vi "Get variant data type name.vi"(8 "error in (no error)":errorcluster, 11 "variant":variant) -> (0 "error out":errorcluster, 3 "resulting string":string)   [LabVIEW 2026, in "TALOS.lvlib"]
uses:
  TALOS.lvlib
  <vilib>/Utility/Data Type/NI_Data Type.lvlib
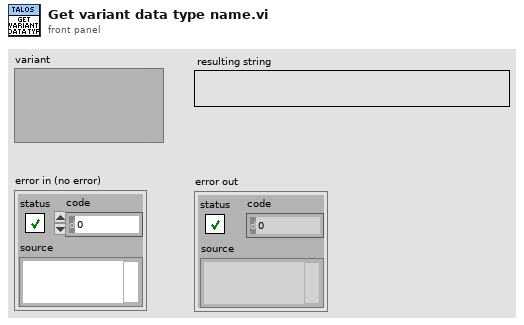
[diagram p1: front panel]
types:
  T1 = typedef "NI_Data Type.lvlib/Data Type.ctl" = enum8{"Invalid Type", "Void", "I8", "I16", "I32", "I64", "U8", "U16", "U32", "U64", "Single Float", "Double Float", "Extended Float", "Single Complex", "Double Complex", "Extended Complex", "Enum U8", "Enum U16", "Enum U32", "Enum U64", "Single Float With Unit", "Double Float With Unit", "Extended Float With Unit", "Single Complex with Unit", "Double Complex with Unit", "Extended Complex with Unit", "Boolean", "String", "Path", "Picture", "Tag", "Array", "Cluster", "Variant", "LV Variant", "Waveform", "Timestamp", "Digital Waveform", "Digital Data", "ExpressData", "Refnum", "External Data", "VI", "Poly VI", "LabVIEW Class Instance", "Fixed Point", "Set Collection", "Map Collection"}
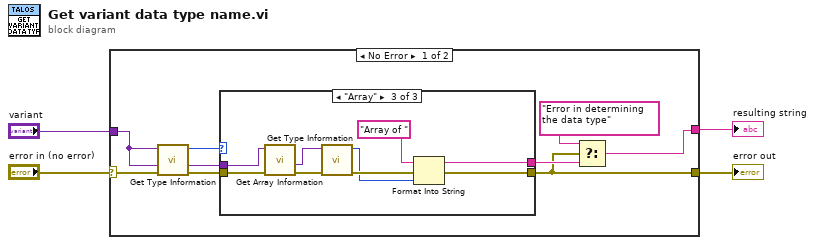
[diagram p0: block diagram]
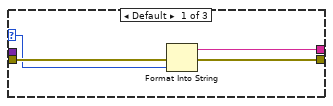
[diagram p2: hidden frame]
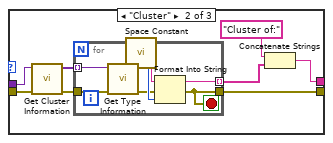
[diagram p3: hidden frame]
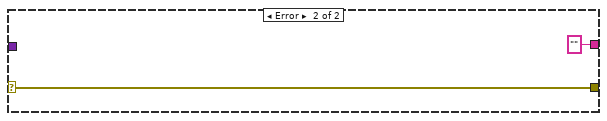
[diagram p4: hidden frame]
diagram:
  n1 = case shown="No Error" "error in (no error)" {
    selector: "error in (no error)" -> [w5 w42]
    tunnel: [w10 "" ("t")] -> w4
    tunnel: [w7 w42] -> w3
    tunnel: "variant" -> [w6 _]
    frame No Error {
      n2 = call <vilib>:"Get Type Information.vi"("error in (no error)"=w5, "variant"=w6) -> ("error out"=w12:errorcluster, "type"=w9:T1)  [unwired: 5 in, 3 out]
      n3 = case shown="\"Array\"" w9 {
        selector: w9 -> [w14 _ _]
        tunnel: w6 -> [_ w24 w39]
        tunnel: w12 -> [w16 w21 w40]
        tunnel: [w13 w20 w33] -> w7
        tunnel: [w15 w17 w32] -> w8
        frame Default {
          n4 = Format Into String(error in=w16, w14) -> (resulting string=w15:string, error out=w13:errorcluster)  [unwired: 2 in]
        }
        frame "Cluster" {
          n5 = call <vilib>:"Get Cluster Information.vi"("error in (no error)"=w21, "variant"=w24) -> ("error out"=w22:errorcluster, "cluster elements"=w23:variant[])  [unwired: 8 in]
          n6 = for {
            tunnel: w23 -> [w31] mode=indexing
            tunnel: w22 -> [w30]
            tunnel: [w27] -> w19 mode=indexing
            tunnel: [w26] -> w20
            stop <- w26 stop-if-true
            n7 = call <vilib>:"Get Type Information.vi"("error in (no error)"=w30, "variant"=w31) -> ("error out"=w28:errorcluster, "type"=w29:T1)  [unwired: 5 in, 3 out]
            n8 = call <vilib>:"Space Constant.vi"() -> ("String"=w25:string)
            n9 = Format Into String(initial string=w25, error in=w28, w29) -> (resulting string=w27:string, error out=w26:errorcluster)  [unwired: 1 in]
          }
          n10 = Concatenate Strings("Cluster of:" ("string"), w19) -> (w17:string)
        }
        frame "Array" {
          n11 = call <vilib>:"Get Array Information.vi"("error in (no error)"=w40, "variant"=w39) -> ("error out"=w38:errorcluster, "array element data type"=w37:variant)  [unwired: 6 in, 2 out]
          n12 = call <vilib>:"Get Type Information.vi"("error in (no error)"=w38, "variant"=w37) -> ("error out"=w36:errorcluster, "type"=w35:T1)  [unwired: 5 in, 3 out]
          n13 = Format Into String(initial string="Array of ", error in=w36, w35) -> (resulting string=w32:string, error out=w33:errorcluster)  [unwired: 1 in]
        }
      }
      n14 = Select(t="Error in determining the data type", s=w7, f=w8) -> (s? t:f=w10:string)
    }
    frame Error {
    }
  }
  "error out" <- w3
  "resulting string" <- w4
